vi "convert_temperature_CCP.vi"(7 "conv_type":enum16{"None", "K2C", "K2F"}(ring), 11 "T_in":dbl) -> (3 "T_out":dbl)   [LabVIEW 2019]
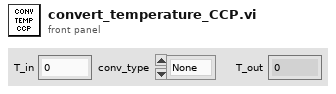
[diagram p1: front panel]
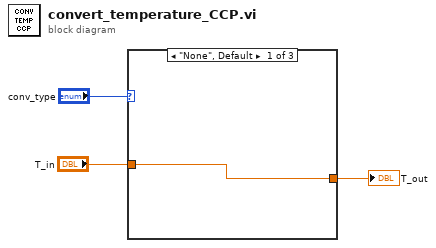
[diagram p0: block diagram]
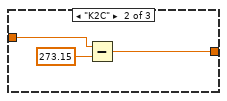
[diagram p2: hidden frame]
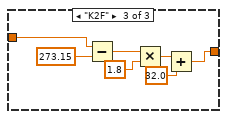
[diagram p3: hidden frame]
diagram:
  n1 = case shown="\"None\", Default" "conv_type" {
    tunnel: "T_in" -> [w4 w7 w13]
    tunnel: [w4 w5 w8] -> w1
    frame "None", Default {
    }
    frame "K2C" {
      n2 = Subtract(x=w7, y=273.15) -> (x-y=w5:dbl)
    }
    frame "K2F" {
      n3 = Subtract(x=w13, y=273.15) -> (x-y=w12:dbl)
      n4 = Multiply(x=w12, y=1.8) -> (x*y=w10:dbl)
      n5 = Add(x=w10, y=32.0) -> (x+y=w8:dbl)
    }
  }
  "T_out" <- w1
